vi "fgv_fgen-visa.vi"() -> ()   [LabVIEW 2021]
uses:
  ctrl/fgen.ctl
panel:
  in  "cmd":T1
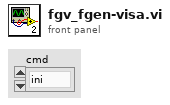
[diagram p1: front panel]
types:
  T1 = typedef "fgen.ctl" = enum16{"ini", "config", "run", "close"}
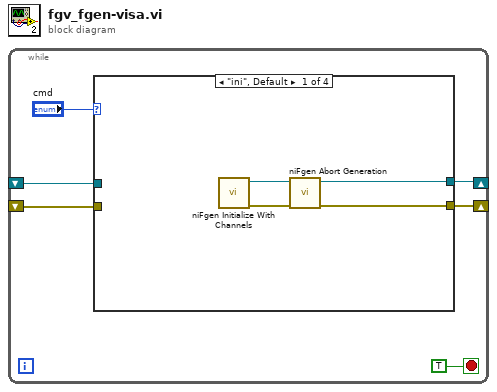
[diagram p0: block diagram]
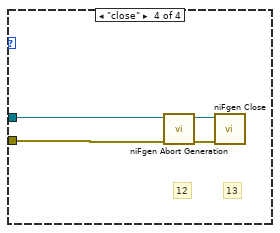
[diagram p4: hidden frame]
diagram:
  n1 = while {
    shift-right: [w3] -> _
    shift-left: _ -> [w2]
    shift-right: [w4] -> _
    shift-left: _ -> [w1]
    stop <- TRUE stop-if-true
    n2 = case shown="\"ini\", Default" "cmd" {
      tunnel: [w8 _ _ _] -> w4
      tunnel: [w7 _ _ _] -> w3
      tunnel: w2 -> [_ _ _ w12]
      tunnel: w1 -> [_ _ _ w11]
      frame "ini", Default {
        n3 = call <instrlib>:"niFgen Initialize With Channels.vi"() -> ("error out"=w10:errorcluster, "Instrument Handle Out"=w9:refnum<k15>)  [unwired: 10 in]
        n4 = call <instrlib>:"niFgen Abort Generation.vi"("error in (no error)"=w10, "Instrument Handle"=w9) -> ("error out"=w8:errorcluster, "Instrument Handle Out"=w7:refnum<k15>)  [unwired: 8 in]
      }
      frame "config" {
      }
      frame "run" {
      }
      frame "close" {
        # "13"
        # "12"
        n5 = call <instrlib>:"niFgen Abort Generation.vi"("error in (no error)"=w11, "Instrument Handle"=w12) -> ("error out"=w13:errorcluster, "Instrument Handle Out"=w14:refnum<k15>)  [unwired: 8 in]
        n6 = call <instrlib>:"niFgen Close.vi"("error in (no error)"=w13, "Instrument Handle"=w14) -> ()  [unwired: 9 in, 1 out]
      }
    }
  }
